vi "Handle Command.vi"(8 "error in (no error)":errorcluster, 9 "Value":bool, 11 "Valve in":refnum<class "DigitalControl.lvclass">) -> (0 "error out":errorcluster, 3 "Valve out":refnum<class "DigitalControl.lvclass">)   [LabVIEW 2020, in "VolatusControl.lvlib" / "DigitalControl.lvclass"]
uses:
  DigitalControl.lvclass
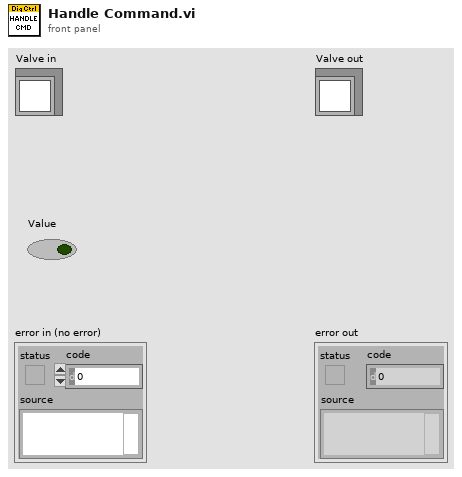
[diagram p1: front panel]
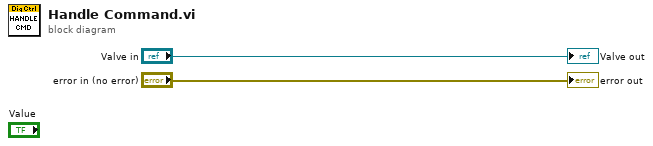
[diagram p0: block diagram]
diagram:
  "error out" <- "error in (no error)"
  "Valve out" <- "Valve in"
